vi "Add.vi"(10 "Y":string="333333333444444444", 11 "X":string="222222222333333333") -> (3 "Sum":string)   [LabVIEW 2021, in "Large Number Operation Engine.lvlib"]
uses:
  Large Number Operation Engine.lvlib
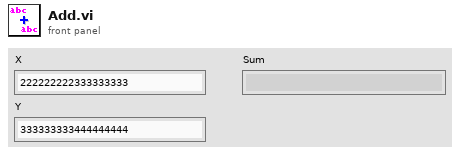
[diagram p1: front panel]
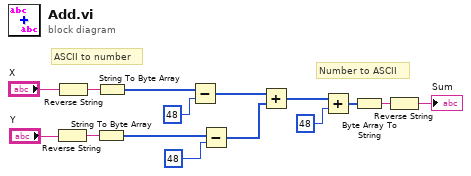
[diagram p0: block diagram]
diagram:
  # "Number to ASCII"
  # "ASCII to number"
  n1 = Reverse String(1:"Y") -> (0:w13:string)
  n2 = Reverse String(1:"X") -> (0:w14:string)
  n3 = String To Byte Array(string=w13) -> (unsigned byte array=w8:u8[])
  n4 = String To Byte Array(string=w14) -> (unsigned byte array=w9:u8[])
  n5 = Subtract(x=w9, y=u8 48) -> (x-y=w2:u8[])
  n6 = Subtract(x=w8, y=u8 48) -> (x-y=w1:u8[])
  n7 = Add(x=w2, y=w1) -> (x+y=w4:u8[])
  n8 = Add(x=w4, y=u8 48) -> (x+y=w7:u8[])
  n9 = Byte Array To String(unsigned byte array=w7) -> (string=w11:string)
  n10 = Reverse String(1:w11) -> (0:→"Sum":string)
